vi "Search ID string array.vi"(7 "With lower case ?":bool, 10 "Input String":string, 11 "String Array":string[](array[string])) -> (2 "Match String":string, 3 "String found ?":bool)   [LabVIEW 2017]
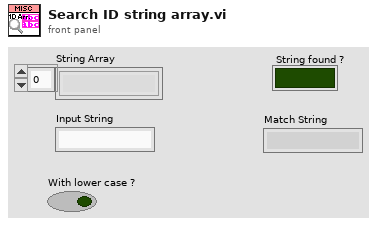
[diagram p1: front panel]
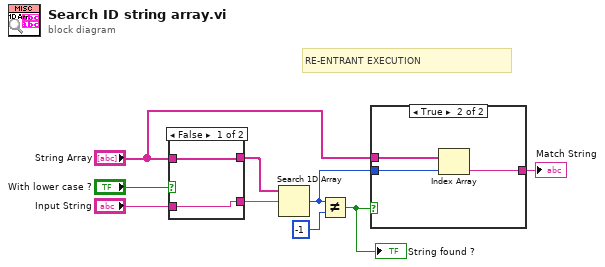
[diagram p0: block diagram]
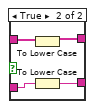
[diagram p2: hidden frame]
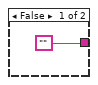
[diagram p3: hidden frame]
diagram:
  # "RE-ENTRANT EXECUTION"
  n1 = case shown="False" "With lower case ?" {
    tunnel: "String Array" -> [w11 w13]
    tunnel: [w11 w14] -> w5
    tunnel: "Input String" -> [w10 w12]
    tunnel: [w10 w15] -> w3
    frame False {
    }
    frame True {
      n2 = To Lower Case(string=w13) -> (all lower case string=w14:string[])
      n3 = To Lower Case(string=w12) -> (all lower case string=w15:string)
    }
  }
  n4 = Search 1D Array(1D array=w5, element=w3) -> (index of element=w7:i32)  [unwired: 1 in]
  n5 = Not Equal?(x=w7, y=-1) -> (x != y?=w8:bool)
  "String found ?" <- w8
  n6 = case shown="True" w8 {
    tunnel: w7 -> [_ w19]
    tunnel: ["" w18] -> w6
    tunnel: "String Array" -> [_ w17]
    frame False {
    }
    frame True {
      n7 = Index Array(array=w17, index=w19) -> (element=w18:string)
    }
  }
  "Match String" <- w6
